vi "S-Curve Goal Calc.vi"(4 "v_f":dbl, 6 "v_i":dbl, 7 "x":dbl, 8 "t":dbl, 9 "j":dbl, 10 "a":dbl, 11 "v":dbl) -> (3 "goal":dbl)   [LabVIEW 2020]
uses:
  sub-vi/Sigmoid.vi
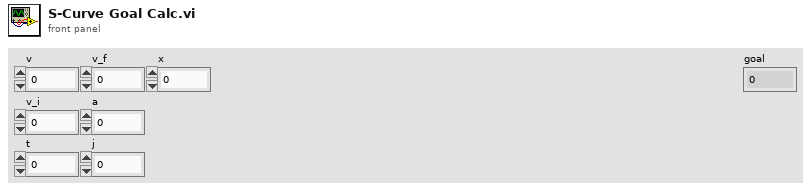
[diagram p1: front panel]
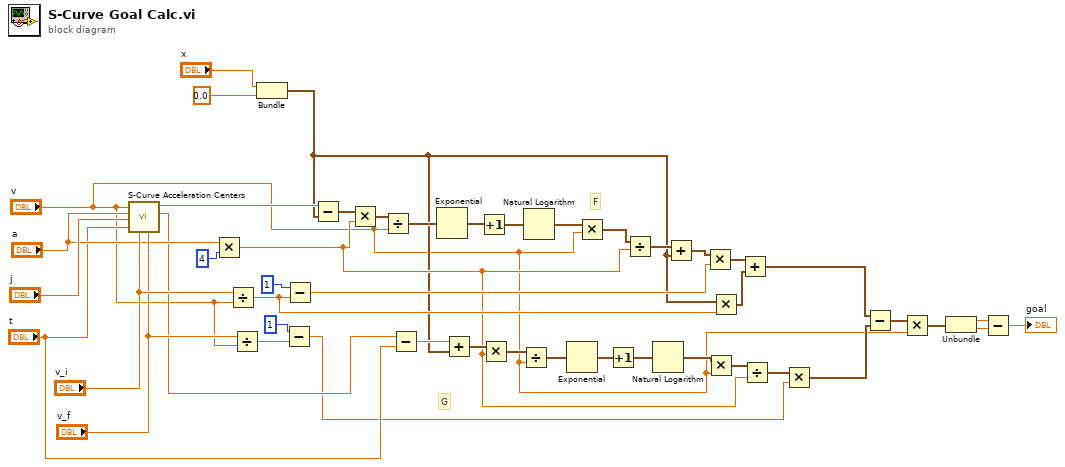
[diagram p0: block diagram]
diagram:
  # "F"
  # "G"
  n1 = call "S-Curve Acceleration Centers.vi"("v_f"="v_f", "v_i"="v_i", "t"="t", "j"="j", "a"="a", "v"="v") -> ("c2"=w24:dbl, "c1"=w38:dbl)  [unwired: 4 in]
  n2 = Multiply(x="a", y=4 ("x")) -> (x*y=w14:dbl)
  n3 = Divide(x="v_i", y="v") -> (x/y=w28:dbl)
  n4 = Divide(x="v_f", y="v") -> (x/y=w42:dbl)
  n5 = Bundle("x"="x", "x"=0.0) -> (w11:cluster{"x":dbl, "x":dbl})  [unwired: 1 in]
  n6 = Subtract(x=1, y=w42) -> (x-y=w12:dbl)
  n7 = Subtract(x=1, y=w28) -> (x-y=w30:dbl)
  n8 = Subtract(x=w38, y=w11) -> (x-y=w37:cluster{"x":dbl, "x":dbl})
  n9 = Multiply(x=w37, y=w14) -> (x*y=w36:cluster{"x":dbl, "x":dbl})
  n10 = Divide(x=w36, y="v") -> (x/y=w35:cluster{"x":dbl, "x":dbl})
  n11 = Subtract(x=w24, y="t") -> (x-y=w22:dbl)
  n12 = Exponential(1:w35) -> (0:w34:cluster{"x":dbl, "x":dbl})
  n13 = Add(x=w22, y=w11) -> (x+y=w21:cluster{"x":dbl, "x":dbl})
  n14 = Increment(x=w34) -> (x+1=w26:cluster{"x":dbl, "x":dbl})
  n15 = Multiply(x=w21, y=w14) -> (x*y=w20:cluster{"x":dbl, "x":dbl})
  n16 = Divide(x=w20, y="v") -> (x/y=w19:cluster{"x":dbl, "x":dbl})
  n17 = Natural Logarithm(1:w26) -> (0:w25:cluster{"x":dbl, "x":dbl})
  n18 = Exponential(1:w19) -> (0:w18:cluster{"x":dbl, "x":dbl})
  n19 = Multiply(x=w25, y="v") -> (x*y=w33:cluster{"x":dbl, "x":dbl})
  n20 = Increment(x=w18) -> (x+1=w17:cluster{"x":dbl, "x":dbl})
  n21 = Divide(x=w33, y=w14) -> (x/y=w32:cluster{"x":dbl, "x":dbl})
  n22 = Natural Logarithm(1:w17) -> (0:w16:cluster{"x":dbl, "x":dbl})
  n23 = Add(x=w32, y=w11) -> (x+y=w31:cluster{"x":dbl, "x":dbl})
  n24 = Multiply(x=w31, y=w30) -> (x*y=w29:cluster{"x":dbl, "x":dbl})
  n25 = Multiply(x=w16, y="v") -> (x*y=w15:cluster{"x":dbl, "x":dbl})
  n26 = Multiply(x=w11, y=w28) -> (x*y=w27:cluster{"x":dbl, "x":dbl})
  n27 = Add(x=w29, y=w27) -> (x+y=w10:cluster{"x":dbl, "x":dbl})
  n28 = Divide(x=w15, y=w14) -> (x/y=w13:cluster{"x":dbl, "x":dbl})
  n29 = Multiply(x=w13, y=w12) -> (x*y=w9:cluster{"x":dbl, "x":dbl})
  n30 = Subtract(x=w10, y=w9) -> (x-y=w8:cluster{"x":dbl, "x":dbl})
  n31 = Multiply(x=w8, y="v") -> (x*y=w6:cluster{"x":dbl, "x":dbl})
  n32 = Unbundle(w6) -> ("x"=w5:dbl, "x"=w4:dbl)
  n33 = Subtract(x=w5, y=w4) -> (x-y=→"goal":dbl)
